vi "CoMP-S Mechanism - Rotation Verification.vi"(8 "error in (no error)":errorcluster, 11 "String":string) -> (0 "error out":errorcluster)   [LabVIEW 2014]
panel:
  out "ROTATION:":string
  in  "OK":bool
  # "If ROTATION status is equal to current position press OK"
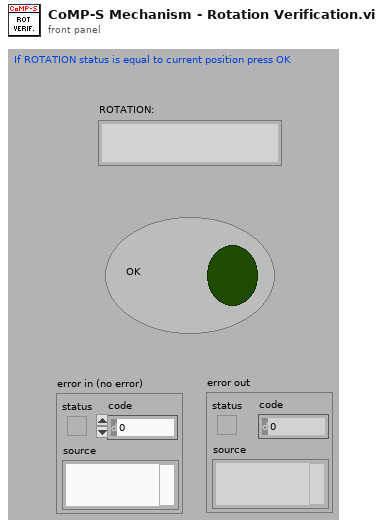
[diagram p1: front panel]
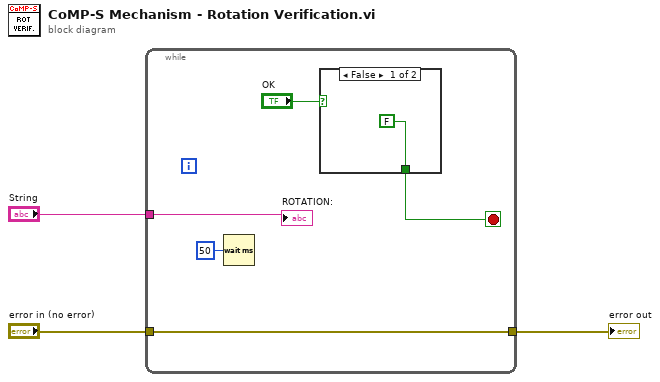
[diagram p0: block diagram]
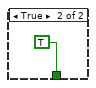
[diagram p2: hidden frame]
diagram:
  n1 = while {
    tunnel: "String" -> [w5]
    tunnel: "error in (no error)" -> [w4]
    tunnel: [w4] -> w2
    stop <- w6 stop-if-true
    n2 = Wait (ms)(milliseconds to wait=u32 50) -> ()  [unwired: 1 out]
    n3 = case shown="False" "OK" {
      tunnel: [FALSE TRUE] -> w6
      frame False {
      }
      frame True {
      }
    }
    "ROTATION:" <- w5
  }
  "error out" <- w2
